vi "InputSecondsToMs.vi"(0 "lower limit":dbl, 2 "description":string, 5 "value (s)":dbl, 7 "upper limit":dbl=999.999, 11 "error in (no error)":errorcluster, 13 "tolerance (fractional)":dbl=0.1) -> (4 "result (ms)":i64, 15 "error out":errorcluster)   [LabVIEW 2014]
doc: "Use this template to build a VI to use as a subVI."
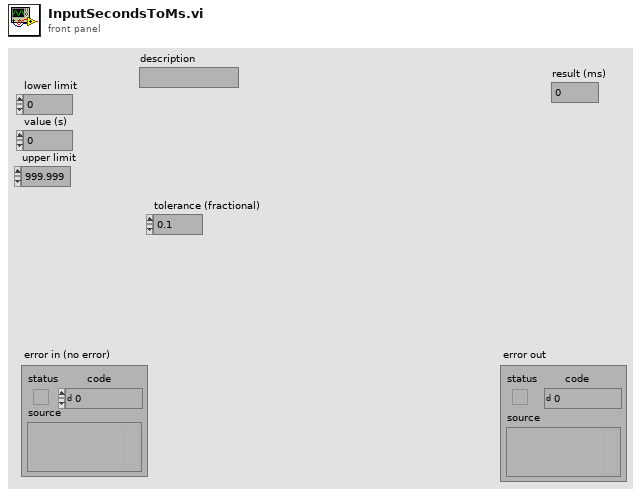
[diagram p1: front panel]
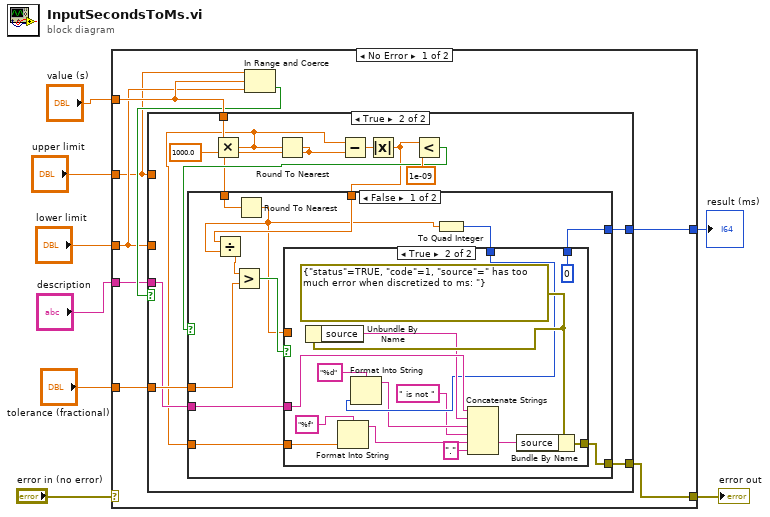
[diagram p0: block diagram]
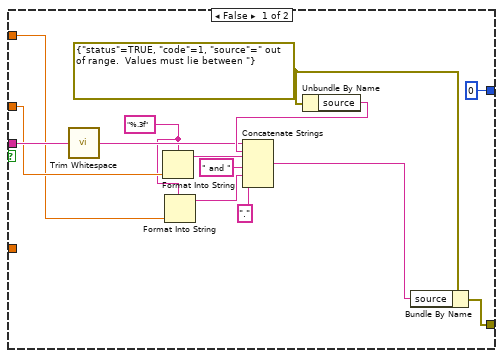
[diagram p2: hidden frame]
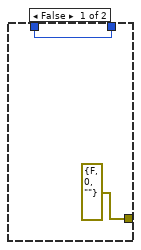
[diagram p3: hidden frame]
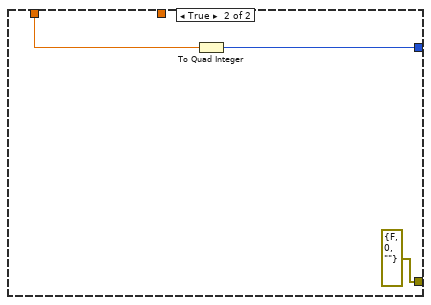
[diagram p4: hidden frame]
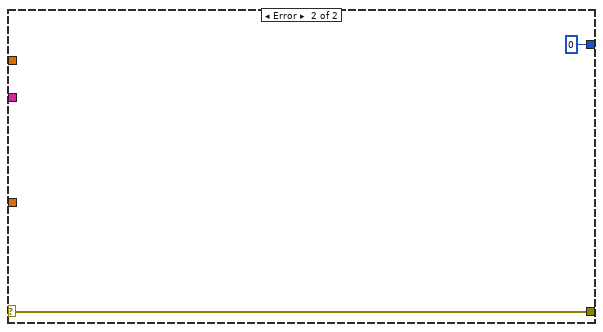
[diagram p5: hidden frame]
diagram:
  n1 = case shown="No Error" "error in (no error)" {
    selector: "error in (no error)" -> [_ w74]
    tunnel: [w14 w74] -> w7
    tunnel: "value (s)" -> [w16 _]
    tunnel: "upper limit" -> [w11 _]
    tunnel: "lower limit" -> [w12 _]
    tunnel: "description" -> [w13 _]
    tunnel: [w10 i64 0] -> w1
    tunnel: "tolerance (fractional)" -> [w9 _]
    frame No Error {
      n2 = In Range and Coerce(upper limit=w11, x=w16, lower limit=w12) -> (In Range?=w15:bool)  [unwired: 1 out]
      n3 = case shown="True" w15 {
        tunnel: w16 -> [_ w41]
        tunnel: [w30 w38] -> w14
        tunnel: w13 -> [w28 w32]
        tunnel: w12 -> [w25 _]
        tunnel: w11 -> [w21 _]
        tunnel: [i64 0 w35] -> w10
        tunnel: w9 -> [_ w33]
        frame False {
          w22 = "%.3f" ("format string")
          w29 = errorcluster {"status"=TRUE, "code"=1, "source"=" out of range.  Values must lie between "} ("error constant")
          n4 = call <vilib>:"Trim Whitespace.vi"("string"=w28) -> ("trimmed string"=w26:string)  [unwired: 1 in]
          n5 = Format Into String(format string=w22, w25) -> (resulting string=w24:string)  [unwired: 2 in, 1 out]
          n6 = Format Into String(format string=w22, w21) -> (resulting string=w20:string)  [unwired: 2 in, 1 out]
          n7 = Unbundle By Name(w29) -> ("source"=w27:string)
          n8 = Concatenate Strings(w26, w27, w24, " and " ("string"), w20, "." ("string")) -> (w18:string)
          n9 = Bundle By Name(cluster=w29, "source"=w18) -> (w30:errorcluster)
        }
        frame True {
          n10 = Multiply(x=w41, y=1000.0) -> (x*y=w31:dbl)
          n11 = Round To Nearest(number=w31) -> (nearest integer value=w36:dbl)
          n12 = Subtract(x=w31, y=w36) -> (x-y=w40:dbl)
          n13 = Absolute Value(x=w40) -> (abs(x)=w34:dbl)
          n14 = Less?(x=w34, y=1e-09) -> (x < y?=w37:bool)
          n15 = case shown="False" w37 {
            tunnel: [w48 errorcluster {"status"=FALSE, "code"=0, "source"=""} ("error constant")] -> w38
            tunnel: w36 -> [w53 w71]
            tunnel: [w44 w70] -> w35
            tunnel: w34 -> [w52 _]
            tunnel: w33 -> [w50 _]
            tunnel: w32 -> [w47 _]
            tunnel: w31 -> [w43 _]
            frame False {
              n16 = Round To Nearest(number=w53) -> (nearest integer value=w46:dbl)
              n17 = Divide(x=w52, y=w46) -> (x/y=w51:dbl)
              n18 = Greater?(x=w51, y=w50) -> (0:w49:bool)
              n19 = To Quad Integer(1:w46) -> (0:w45:i64)
              n20 = case shown="True" w49 {
                tunnel: w46 -> [_ _]
                tunnel: [errorcluster {"status"=FALSE, "code"=0, "source"=""} ("error constant") w69] -> w48
                tunnel: w47 -> [_ w66]
                tunnel: w45 -> [w54 w63]
                tunnel: [w54 i64 0] -> w44
                tunnel: w43 -> [_ w59]
                frame False {
                }
                frame True {
                  w68 = errorcluster {"status"=TRUE, "code"=1, "source"=" has too much error when discretized to ms: "} ("error constant")
                  n21 = Unbundle By Name(w68) -> ("source"=w64:string)
                  n22 = Format Into String(format string="%f", w59) -> (resulting string=w57:string)  [unwired: 2 in, 1 out]
                  n23 = Format Into String(format string="%d", w63) -> (resulting string=w61:string)  [unwired: 2 in, 1 out]
                  n24 = Concatenate Strings(w66, w64, w61, " is not " ("string"), w57, "." ("string")) -> (w67:string)
                  n25 = Bundle By Name(cluster=w68, "source"=w67) -> (w69:errorcluster)
                }
              }
            }
            frame True {
              n26 = To Quad Integer(1:w71) -> (0:w70:i64)
            }
          }
        }
      }
    }
    frame Error {
    }
  }
  "error out" <- w7
  "result (ms)" <- w1
